vi "Experiement Dryer Weight Analysis 1.vi"() -> ()   [LabVIEW 2009]
uses:
  <vilib>/Analysis/NI_AALBase.lvlib
panel:
  out "Samples per Capture":i32=100000
  out "Average of Filtered Data":dbl[](graph)=[111.6794692825523, 111.6412698121877, 111.6794692825523, 111.6412698121877, 111.6794692825523, 111.65143087130468, 111.6794692825523, 111.64463136557978, 111.64627394280546, 111.6412698121877, 111.6412698121877, 111.6030703418231, 111.5648708714585, 111.6030703418231, 111.6412698121877, 111.6030703418231, 111.6030703418231, 111.5648708714585, 111.5648708714585, 111.52667140109389, 111.52667140109389, 111.57224336923886, 111.6030703418231, 111.5648708714585, 111.6030703418231, 111.6030703418231, 111.6412698121877, 111.6030703418231, 111.6030703418231, 111.5648708714585, 111.5648708714585, 111.6030703418231, 111.6412698121877, 111.5648708714585, 111.52667140109389, 111.6412698121877, 111.6030703418231, 111.6030703418231, 111.6030703418231, 111.6030703418231, 111.6030703418231, 111.5648708714585, 111.6030703418231, 111.6412698121877, 111.6412698121877, 111.67297537259032, 111.6030703418231, 111.6412698121877, 111.61647835592107, 111.6030703418231, 111.5648708714585, 111.6030703418231, 111.6412698121877, 111.6794692825523, 111.6412698121877, 111.6794692825523, 111.6794692825523, 111.6412698121877, 111.6412698121877, 111.6794692825523, 111.6412698121877, 111.6412698121877, 111.6412698121877, 111.6412698121877, 111.60731048303357, 111.6412698121877, 111.6399710301953, 111.6794692825523, 111.6794692825523, 111.6412698121877, 111.6794692825523, 111.6412698121877, 111.6412698121877, 111.6412698121877, 111.6412698121877, 111.6412698121877, 111.6412698121877, 111.6412698121877, 111.6412698121877, 111.6412698121877, 111.64535715551672, 111.6794692825523, 111.6794692825523, 111.6412698121877, 111.6412698121877, 111.6412698121877, 111.6412698121877, 111.6412698121877, 111.6412698121877]
  in  "Truncation":i32=49500
  out "Average of each Capture":dbl[](graph)=[111.64851052179532, 111.64237683283888, 111.65399672972909, 111.64005506903011, 111.64765561764857, 111.64399190644589, 111.65078797421846, 111.64282529462096, 111.64338911880354, 111.62927747046145, 111.63858056947404, 111.60055032276317, 111.55681383916921, 111.60186132858607, 111.62947190576561, 111.60956081383277, 111.59281454801963, 111.56337765416197, 111.56017233660367, 111.49904707210504, 111.51104476175716, 111.57164898548001, 111.5839591467997, 111.56182942962809, 111.58169735615941, 111.59000650495312, 111.61693369360783, 111.60967617623326, 111.57363688591778, 111.55710530112809, 111.55870547694167, 111.60341146309347, 111.63175394212519, 111.5611911164783, 111.54096335093612, 111.61736725759647, 111.58926963716979, 111.57790758670454, 111.59042020521717, 111.60719206467546, 111.58135241494203, 111.55544438815664, 111.57899397964171, 111.64012230009796, 111.63811338995149, 111.64588239823424, 111.59423938826423, 111.61500003641798, 111.61144633968996, 111.60148086186125, 111.56845054382639, 111.59183320362595, 111.62159020904527, 111.65453610625063, 111.62049617621403, 111.65818835761219, 111.68548837309766, 111.6352232180237, 111.62477413490016, 111.65364147465469, 111.63144758237287, 111.64094206073199, 111.63650519224913, 111.63017477602031, 111.60934995275635, 111.63017363003621, 111.61380286501675, 111.67833781424011, 111.65024286777636, 111.63227116295393, 111.66217600032356, 111.64168313045705, 111.63884681978249, 111.62887790400144, 111.62914377231517, 111.64275004166434, 111.64165982878013, 111.63475374653292, 111.62555264010619, 111.6223469405532, 111.6441286605498, 111.64846200846796, 111.65565229477468, 111.63911345208562, 111.64037938253351, 111.64083433822556, 111.64025447026542, 111.63429955483028, 111.62433331301216]
  out "Num Captures":i32=89
  out "Total Data, Weight":waveform(dbl)(graph)={"t0"=timestamp(3400754986.84385 s since 1904-01-01), "dt"=9.999999999999999e-05, "Y"=array[100000 elements], "attributes"=variant("NI_ChannelName"=variant(string "Voltage"), "NI_UnitDescription"=variant(string "lbs"))}
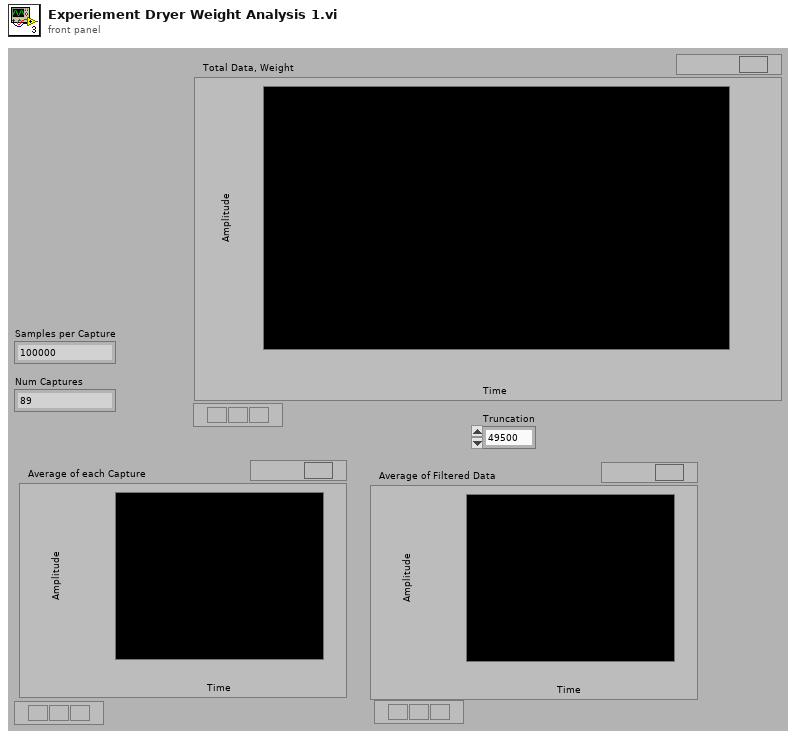
[diagram p1: front panel]
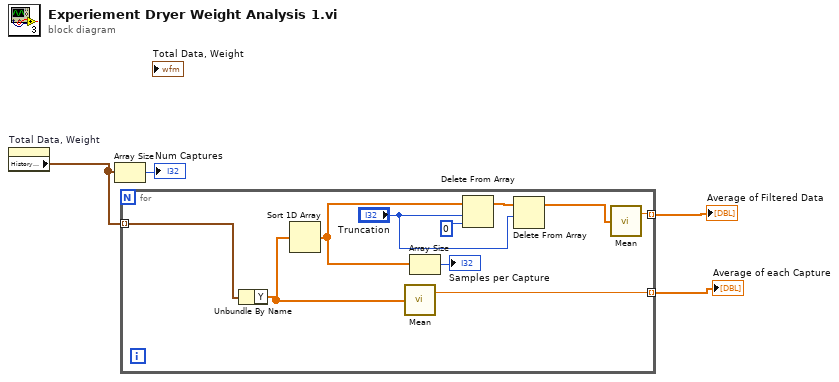
[diagram p0: block diagram]
diagram:
  n1 = property on="Total Data, Weight" class="WFChart (strict)"() -> ("History Data"=w3:waveform(dbl)[])  [unwired: 2 in, 2 out]
  n2 = Array Size(array=w3) -> (size(s)=→"Num Captures":i32)
  n3 = for {
    tunnel: w3 -> [w14] mode=indexing
    tunnel: [w13] -> w2 mode=indexing
    tunnel: [w7] -> w1 mode=indexing
    n4 = Unbundle By Name(w14) -> ("Y"=w12:dbl[])
    n5 = Sort 1D Array(array=w12) -> (sorted array=w5:dbl[])
    n6 = call <vilib>:"Mean.vi"("X"=w12) -> ("mean"=w13:dbl)  [unwired: 1 out]
    n7 = Array Size(array=w5) -> (size(s)=→"Samples per Capture":i32)
    n8 = Delete From Array(array=w5, length="Truncation", index=0) -> (array with subset deleted=w11:dbl[])  [unwired: 1 out]
    n9 = Delete From Array(array=w11, length="Truncation") -> (array with subset deleted=w8:dbl[])  [unwired: 1 in, 1 out]
    n10 = call <vilib>:"Mean.vi"("X"=w8) -> ("mean"=w7:dbl)  [unwired: 1 out]
  }
  "Average of each Capture" <- w2
  "Average of Filtered Data" <- w1
